vi "thermistor_manager.vi"(3 "input valid":bool=TRUE, 4 "V":fxp<+,21,5>, 5 "count":u16) -> (0 "input_index":u16, 1 "temperature":fxp<+/-,32,16>, 2 "output_index":u16)   [LabVIEW 2018]
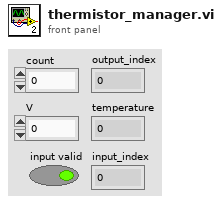
[diagram p1: front panel]
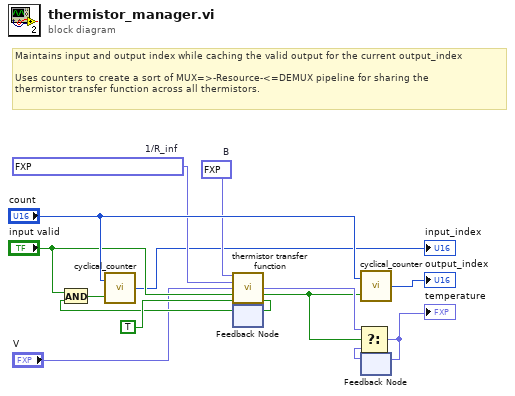
[diagram p0: block diagram]
diagram:
  w11 = fxp<+,32,7> 10.047783523797989  # 1/R_inf
  w12 = fxp<+/-,32,16> 3434.0  # B
  # "Maintains input and output index while caching the valid output for the current output_index\n\nUses counters to create a sort of MUX=>-Resource-<=DEMUX pipeline for sharing the\nthermistor transfer function across all thermistors."
  n1 = call "thermistor transfer function.vi"("B"=w12, "1/R_inf"=w11, "V"="V", "input valid"="input valid", "ready for output (T)"=TRUE) -> ("Temperature"=w9:fxp<+/-,32,16>, "output valid"=w8:bool, "ready for input"=w15:bool)  [unwired: 8 in]
  n2 = feedback #1() -> (w3:bool)  [unwired: 1 in]
  n3 = And(x="input valid", y=w3) -> (x .and. y?=w4:bool)
  n4 = call "cyclical_counter.vi"("Enable"=w4, "Mod"="count") -> ("Count"=→"input_index":u16)
  n5 = feedback-in #1(w15) -> ()
  n6 = call "cyclical_counter.vi"("Enable"=w8, "Mod"="count") -> ("Count"=→"output_index":u16)
  n7 = feedback #2() -> (w6:fxp<+/-,32,16>)  [unwired: 1 in]
  n8 = Select(t=w9, s=w8, f=w6) -> (s? t:f=w7:fxp<+/-,32,16>)
  "temperature" <- w7
  n9 = feedback-in #2(w7) -> ()
